vi "Specify range command.vi"(8 "error in (no error)":errorcluster, 10 "Range":T1, 11 "VISA resource name":refnum<visa-resource-name>="GPIB0::21::INSTR") -> (0 "error out":errorcluster, 3 "VISA resource name out":refnum<visa-resource-name>)   [LabVIEW 2009]
uses:
  Range control watts.ctl
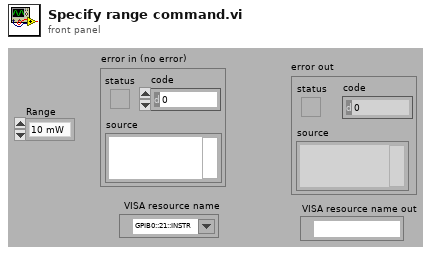
[diagram p1: front panel]
types:
  T1 = typedef "Range control watts.ctl" = enum16{"10 mW", "1 mW", "100 uW", "10 uW", "1 uW", "100 nW", "10 nW", "1 nW", "100 pW", "10 pW"}
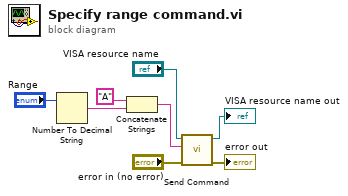
[diagram p0: block diagram]
diagram:
  n1 = Number To Decimal String(number="Range") -> (decimal integer string=w3:string)  [unwired: 1 in]
  n2 = Concatenate Strings("A" ("string"), w3) -> (w1:string)
  n3 = call "Send Command.vi"("error in (no error)"="error in (no error)", "write buffer"=w1, "VISA resource name"="VISA resource name") -> ("error out"=→"error out":errorcluster, "VISA resource name out"=→"VISA resource name out":refnum<visa-resource-name>)  [unwired: 7 in]
